vi "Login_Screen.vi"(8 "error constant":errorcluster) -> (0 "error constant 2":errorcluster, 1 "Operator Name 2":string, 2 "Admin?":bool)   [LabVIEW 2024, in "Launcher_DTU.lvlib"]
uses:
  Launcher_DTU.lvlib
  Login_ctrl.ctl
  Global 1.vi
panel:
  in  "Close":bool
  in  "Del name":bool
  in  "Add name":bool
  in  "Login":bool
  in  "Operator Name":string(combo)
  in  "Log member":enum16{"Admin", "Engineering_Mode", "Operator"}(ring)
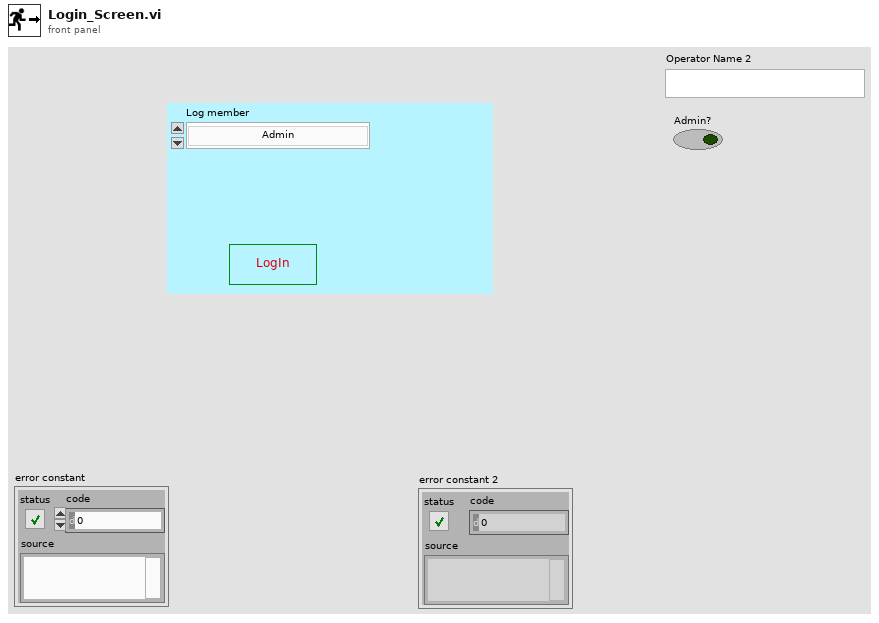
[diagram p1: front panel]
types:
  T1 = typedef "Login_ctrl.ctl" = enum16{"Init", "Poll", "Add_OP", "DEL_OP", "Save_op", "Read_op_details", "Exit"}
  T2 = cluster{"Operator name":string, "Operator path":path, "Op_name_pW":cluster{"Operator name":string, "Password":string}[], "Login":bool, "Log member":enum16{"Admin", "Engineering_Mode", "Operator"}}
  T3 = cluster{"OP_name":cluster{"Operator name":string, "Password":string}[]}
  T4 = cluster{"Operator name":string, "Password":string}[]
  T5 = cluster{"Operator name":string, "Password":string}
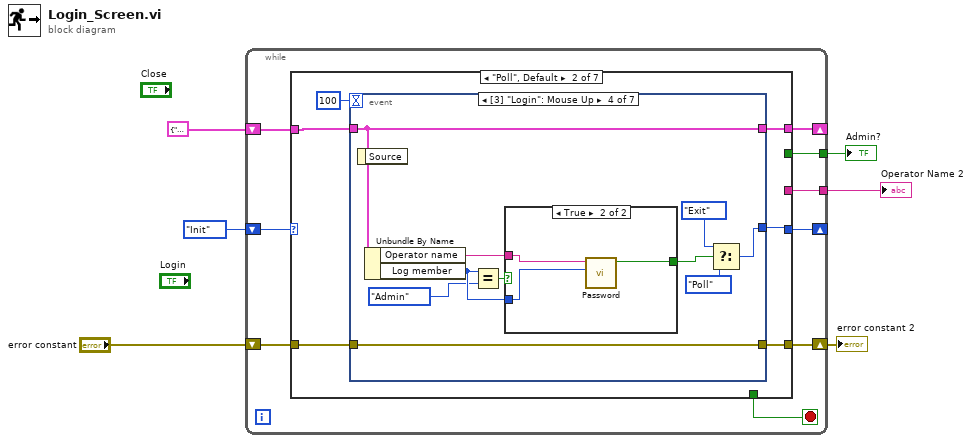
[diagram p0: block diagram]
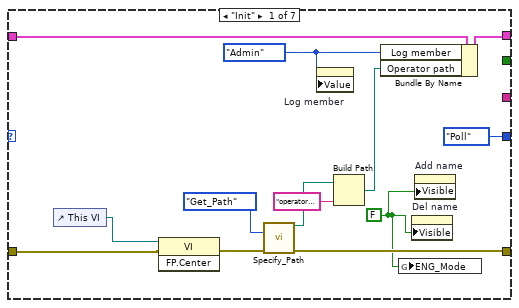
[diagram p2: hidden frame]
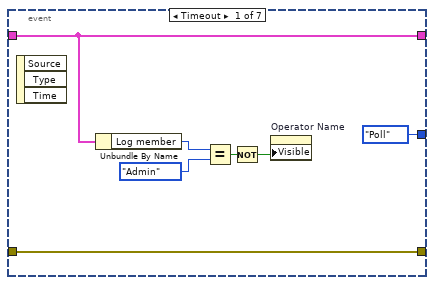
[diagram p3: hidden frame]
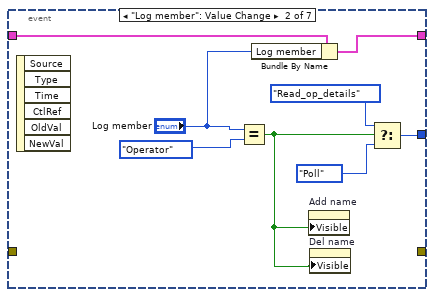
[diagram p4: hidden frame]
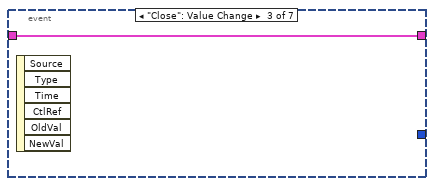
[diagram p5: hidden frame]
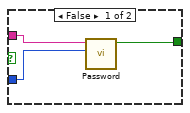
[diagram p6: hidden frame]
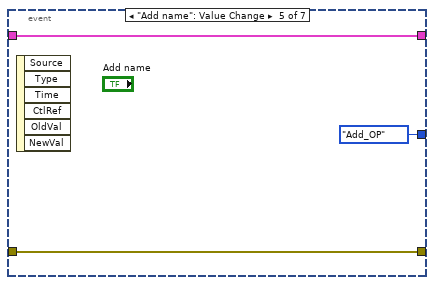
[diagram p7: hidden frame]
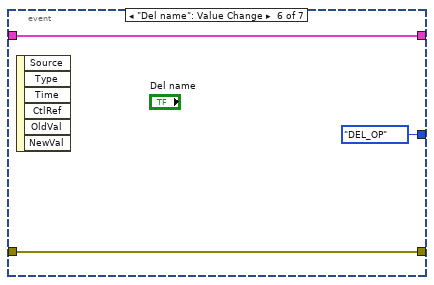
[diagram p8: hidden frame]
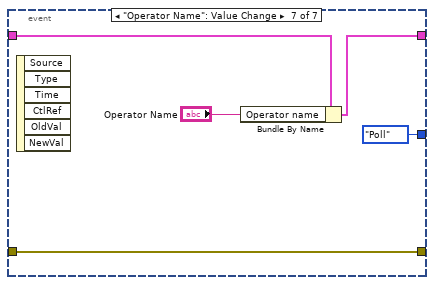
[diagram p9: hidden frame]
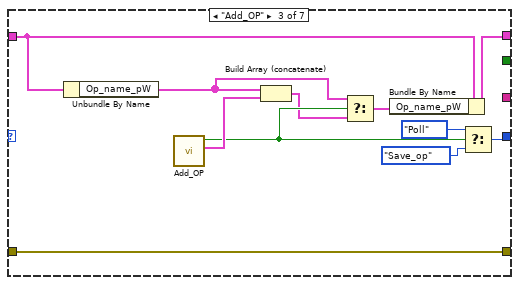
[diagram p10: hidden frame]
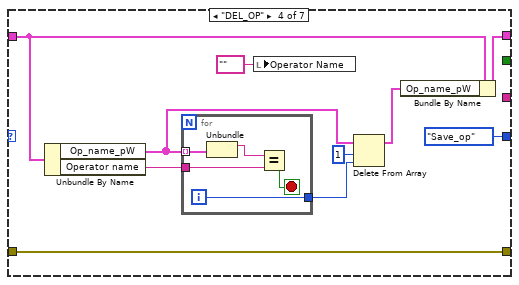
[diagram p11: hidden frame]
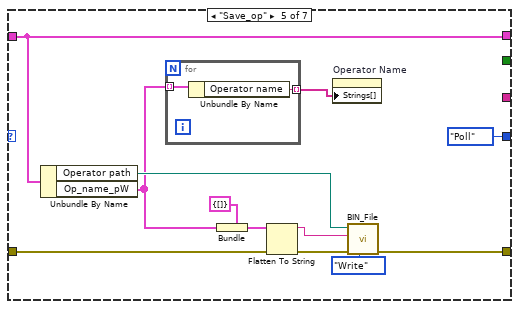
[diagram p12: hidden frame]
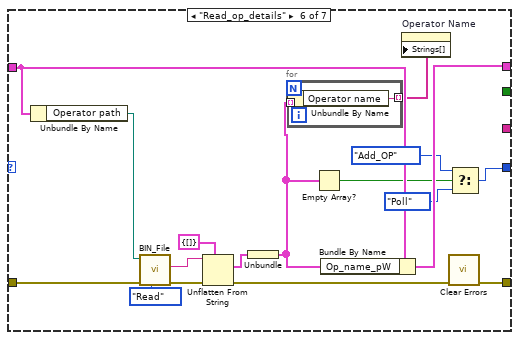
[diagram p13: hidden frame]
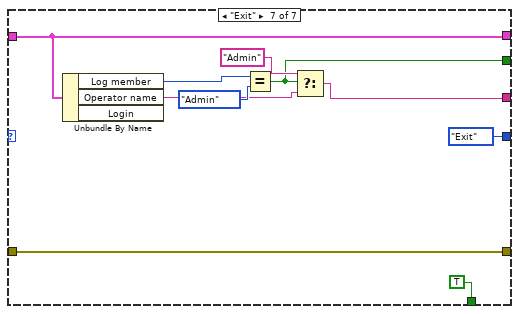
[diagram p14: hidden frame]
diagram:
  n1 = while {
    shift-right: [w12] -> _
    shift-left: T2 {"Operator name"="", "Operator path"=path "", "Op_name_pW"=[], "Login"=TRUE, "Log member"=enum."Admin"} -> [w15]
    shift-right: [w13] -> w2
    shift-left: "error constant" -> [w14]
    tunnel: [w10] -> w4
    tunnel: [w9] -> w3
    shift-right: [w7] -> _
    shift-left: Login_ctrl."Init" -> [w8]
    stop <- w11 stop-if-true
    n2 = case shown="\"Poll\", Default" w8 {
      tunnel: w15 -> [w28 w32 w87 w96 w113 w133 w144]
      tunnel: w14 -> [w26 w34 w88 w98 w115 w134 w146]
      tunnel: [w22 w33 w88 w98 w112 w120 w146] -> w13
      tunnel: [w27 w31 w79 w91 w113 w127 w144] -> w12
      tunnel: [_ _ _ _ _ _ TRUE] -> w11
      tunnel: [_ _ _ _ _ _ w139] -> w10
      tunnel: [_ _ _ _ _ _ w138] -> w9
      tunnel: [Login_ctrl."Poll" w29 w82 Login_ctrl."Save_op" ("f") Login_ctrl."Poll" ("f") w125 Login_ctrl."Exit" ("f")] -> w7
      frame "Init" {
        w17 = enum16{"Admin", "Engineering_Mode", "Operator"}."Admin" ("Log member")
        w16 = FALSE
        n3 = control-ref of="This VI"() -> (w24:refnum<vi>)
        n4 = invoke class="VI" method="FP.Center"(reference=w24, error in=w26) -> (error out=w25:errorcluster)  [unwired: 1 in, 2 out]
        n5 = call "Specify_Path.vi"("Path_Enum"=enum16{"Find_Path", "Get_Path"}."Get_Path", "error in (no error)"=w25) -> ("Configurations"=w20:path, "error out"=w22:errorcluster)  [unwired: 6 in, 6 out]
        n6 = property on="Log member" class="Enum (strict)"("Value"=w17) -> ()  [unwired: 2 in, 2 out]
        n7 = Build Path(base path=w20, name or relative path="operator_info.bin") -> (appended path=w18:path)
        n8 = Bundle By Name(cluster=w28, "Log member"=w17, "Operator path"=w18) -> (w27:T2)
        n9 = global write "Global 1.vi" "ENG_Mode"(w16) -> ()
        n10 = property on="Del name" class="Bool"("Visible"=w16) -> ()  [unwired: 2 in, 2 out]
        n11 = property on="Add name" class="Bool"("Visible"=w16) -> ()  [unwired: 2 in, 2 out]
      }
      frame "Poll", Default {
        n12 = event shown="[3] \"Login\": Mouse Up" {
          selector: _ -> [_ _ _ _ _ _ _]
          dyn-events: _ -> [_ _ _ _ _ _ _]
          timeout: 100 -> [_ _ _ _ _ _ _]
          tunnel: [w41 _ _ w60 w69 w71 w76] -> w33
          tunnel: w34 -> [w41 _ _ w60 w69 w71 w76]
          tunnel: [w40 w48 w50 w59 w67 w72 w75] -> w31
          tunnel: w32 -> [w40 w49 w50 w59 w67 w72 w77]
          tunnel: [Login_ctrl."Poll" ("f") w44 _ w54 Login_ctrl."Add_OP" ("f") Login_ctrl."DEL_OP" ("f") Login_ctrl."Poll" ("f")] -> w29
          event Timeout {
            n13 = event-data() -> ()  [unwired: 1 in, 3 out]
            n14 = Unbundle By Name(w40) -> ("Log member"=w39:enum16{"Admin", "Engineering_Mode", "Operator"})
            n15 = Equal?(x=w39, y=enum16{"Admin", "Operator"}."Admin" ("Log member")) -> (x = y?=w37:bool)
            n16 = Not(x=w37) -> (.not. x?=w36:bool)
            n17 = property on="Operator Name" class="CmbBox"("Visible"=w36) -> ()  [unwired: 2 in, 2 out]
          }
          event "Log member": Value Change {
            n18 = event-data() -> ()  [unwired: 1 in, 6 out]
            n19 = Equal?(x="Log member", y=enum16{"Admin", "Engineering_Mode", "Operator"}."Operator" ("Log member")) -> (x = y?=w43:bool)
            n20 = Bundle By Name(cluster=w49, "Log member"="Log member") -> (w48:T2)
            n21 = property on="Add name" class="Bool"("Visible"=w43) -> ()  [unwired: 2 in, 2 out]
            n22 = property on="Del name" class="Bool"("Visible"=w43) -> ()  [unwired: 2 in, 2 out]
            n23 = Select(t=Login_ctrl."Read_op_details", s=w43, f=Login_ctrl."Poll") -> (s? t:f=w44:T1)
          }
          event "Close": Value Change {
            n24 = event-data() -> ()  [unwired: 1 in, 6 out]
          }
          event "Login": Mouse Up {
            n25 = event-data() -> ()  [unwired: 1 in, 1 out]
            n26 = Unbundle By Name(w59) -> ("Operator name"=w53:string, "Log member"=w52:enum16{"Admin", "Engineering_Mode", "Operator"})
            n27 = Equal?(x=w52, y=enum16{"Admin", "Engineering_Mode", "Operator"}."Admin" ("Log member")) -> (x = y?=w58:bool)
            n28 = case shown="True" w58 {
              tunnel: [w61 w66] -> w57
              tunnel: w53 -> [w63 w65]
              tunnel: w52 -> [w62 w64]
              frame False {
                n29 = call "Password.vi"("Log member"=w62, "Op_name"=w63) -> ("Correct"=w61:bool)  [unwired: 9 in]
              }
              frame True {
                n30 = call "Password.vi"("Log member"=w64, "Op_name"=w65) -> ("Correct"=w66:bool)  [unwired: 9 in]
              }
            }
            n31 = Select(t=Login_ctrl."Exit", s=w57, f=Login_ctrl."Poll") -> (s? t:f=w54:T1)
          }
          event "Add name": Value Change {
            n32 = event-data() -> ()  [unwired: 1 in, 6 out]
          }
          event "Del name": Value Change {
            n33 = event-data() -> ()  [unwired: 1 in, 6 out]
          }
          event "Operator Name": Value Change {
            n34 = event-data() -> ()  [unwired: 1 in, 6 out]
            n35 = Bundle By Name(cluster=w77, "Operator name"="Operator Name") -> (w75:T2)
          }
        }
      }
      frame "Add_OP" {
        n36 = Unbundle By Name(w87) -> ("Op_name_pW"=w81:T4)
        n37 = call "Add_OP.vi"() -> ("ADD/OP"=w86:T5, "Cancel 2"=w84:bool)  [unwired: 10 in]
        n38 = Build Array (concatenate)(w81, w86) -> (w80:T4)
        n39 = Select(t=w81, s=w84, f=w80) -> (s? t:f=w78:T4)
        n40 = Bundle By Name(cluster=w87, "Op_name_pW"=w78) -> (w79:T2)
        n41 = Select(t=Login_ctrl."Poll", s=w84, f=Login_ctrl."Save_op") -> (s? t:f=w82:T1)
      }
      frame "DEL_OP" {
        n42 = Unbundle By Name(w96) -> ("Op_name_pW"=w94:T4, "Operator name"=w95:string)
        n43 = for {
          tunnel: w94 -> [w103] mode=indexing
          tunnel: w95 -> [w102]
          tunnel: [w99] -> w93
          i -> [w99]
          stop <- w100 stop-if-true
          n44 = Unbundle(w103) -> ("Operator name"=w101:string)  [unwired: 1 out]
          n45 = Equal?(x=w101, y=w102) -> (x = y?=w100:bool)
        }
        n46 = local write "Operator Name"("" ("Operator Name")) -> ()
        n47 = Delete From Array(array=w94, length=1, index=w93) -> (array with subset deleted=w90:T4)  [unwired: 1 out]
        n48 = Bundle By Name(cluster=w96, "Op_name_pW"=w90) -> (w91:T2)
      }
      frame "Save_op" {
        n49 = Unbundle By Name(w113) -> ("Operator path"=w111:path, "Op_name_pW"=w105:T4)
        n50 = for {
          tunnel: w105 -> [w117] mode=indexing
          tunnel: [w116] -> w104 mode=indexing
          n51 = Unbundle By Name(w117) -> ("Operator name"=w116:string)
        }
        n52 = Bundle(cluster=T3 {"OP_name"=[]}, "OP_name"=w105) -> (w106:T3)
        n53 = Flatten To String(anything=w106, error in (no error)=w115) -> (data string=w108:string, error out=w109:errorcluster)  [unwired: 2 in, 1 out]
        n54 = property on="Operator Name" class="CmbBox"("Strings[]"=w104) -> ()  [unwired: 2 in, 2 out]
        n55 = call "BIN_File.vi"("Enum"=enum16{"Read", "Write"}."Write", "error in"=w109, "Data"=w108, "Path"=w111) -> ("error out"=w112:errorcluster)  [unwired: 6 in, 1 out]
      }
      frame "Read_op_details" {
        n56 = Unbundle By Name(w133) -> ("Operator path"=w132:path)
        n57 = call "BIN_File.vi"("Enum"=enum16{"Read", "Write"}."Read", "error in"=w134, "Path"=w132) -> ("error out"=w129:errorcluster, "data out"=w130:string)  [unwired: 7 in]
        n58 = Unflatten From String(type=T3 {"OP_name"=[]}, binary string=w130, error in (no error)=w129) -> (value=w121:T3, error out=w128:errorcluster)  [unwired: 2 in, 1 out]
        n59 = Unbundle(w121) -> ("OP_name"=w119:T4)
        n60 = for {
          tunnel: w119 -> [w136] mode=indexing
          tunnel: [w135] -> w118 mode=indexing
          n61 = Unbundle By Name(w136) -> ("Operator name"=w135:string)
        }
        n62 = Empty Array?(array=w119) -> (empty?=w124:bool)
        n63 = Bundle By Name(cluster=w133, "Op_name_pW"=w119) -> (w127:T2)
        n64 = property on="Operator Name" class="CmbBox"("Strings[]"=w118) -> ()  [unwired: 2 in, 2 out]
        n65 = call <vilib>:"Clear Errors.vi"("error in (no error)"=w128) -> ("error out"=w120:errorcluster)  [unwired: 5 in, 1 out]
        n66 = Select(t=Login_ctrl."Add_OP", s=w124, f=Login_ctrl."Poll") -> (s? t:f=w125:T1)
      }
      frame "Exit" {
        n67 = Unbundle By Name(w144) -> ("Log member"=w142:enum16{"Admin", "Engineering_Mode", "Operator"}, "Operator name"=w140:string)  [unwired: 1 out]
        n68 = Equal?(x=w142, y=enum16{"Admin", "Operator"}."Admin" ("Log member")) -> (x = y?=w138:bool)
        n69 = Select(t="Admin", s=w138, f=w140) -> (s? t:f=w139:string)
      }
    }
  }
  "Operator Name 2" <- w4
  "Admin?" <- w3
  "error constant 2" <- w2
